vi "CRYRecall Editor.vi"() -> ()   [LabVIEW 2013]
uses:
  <vilib>/Utility/miscctls.llb/LVBoundsTypeDef.ctl
  Typedef Control/CRYRecall Cluster.ctl
  CRYProject/CRYProject Editor Global.vi
  CRYMainGlobal.vi
  CRYWindow/SubVI/CRYMain Sub Window Global.vi
  SubVI/CRYRecall Global.vi
  CRYStepSetup/CRYStepSetup Global.vi
panel:
  out "Recall Cluster Bk":T1={"Name"="Test for Signal [L]", "filepath"="Test for Signal [L]", "all or last"=0, "File Path Mode"=0, "Curve Names"=[], "format string"={"dB Format String out"="", "Lin Format String out"=""}, "Template"=[], "Axis"=0, "*.imp Path"=path "", "Filepath option"=0, "ML Value"=0.0, "user defined"="Test for Signal [L]", "Curves Selected?"=[], "Help"="", "Tab Value"=enum."Setting", "Selector"=0, "Use Default"=FALSE} {"Selector" items=["Space", "Underscores", "None"]; "Axis" scale=0.0..2.0; "Template" format="%#.0f"}
  in  "CurLibChange":bool caption="Add Lib"
  in  "Current Row":i32
  out "Auto Path":string
  out "Specify Path":string
  out "Auto Names":string[](array[string])
  out "Specify Names":string[](array[string])
  out "EndFlag":bool
  in  "Add Lib":bool
  in  "AddStep":bool
  in  "Table change":bool=TRUE
  out "Data type":string
  out "Row":u32
  in  "Board Tab":enum32{"Page 1"}(tab)
  in  "Cancel":bool caption="Apply"
  in  "OK":bool caption="Apply"
  in  "Main Tab":enum32{"Setting", "Help"}(tab)
  in  "Selector":i32(ring) caption="选择" items=["空格", "下划线", "无"]
  in  "Use default":bool caption="用户定义"
  in  "Format Value":bool
  out "single val":string
  in  "Select All":bool
  in  "Rename":bool
  in  "Clear2":bool
  in  "Add2":bool
  in  "Value":u16(ring) caption="值" items=["Max FSD Out Stimulus", "采集延迟 [Direct Out 1]", "采集延迟 [Direct Out 1] - P", "unity cal-in sens-in", "CRY33x Mic 1 sens-in", "CRY33x Mic 2 sens-in", "CRY33x Mic 3 sens-in", "CRY33x Mic 4 sens-in", "USB In L sens-in", "USB In R sens-in", "unity cal-out sens-out", "CRY602 Mouth 1 sens-out", "CRY602 Mouth 2 sens-out", "USB Out R sens-out", "Max FSD In [Direct In 1]", "2-采集延迟 [Direct Out 1]"]
  out "Template":string caption="模板"
  in  "User defined":string caption="用户定义"
  in  "Clear1":bool
  in  "Add1":bool
  in  "File Path Mode":u16(slide)
  in  "Recall Curve":u16(slide) caption="调用:"
  out "Recalled Curves":bool caption="调用曲线"
  out "File Path Information":bool caption="文件路径信息"
  in  "Base Path":path caption="基地路径"
  in  "Path Info":u16(slide)
  in  "filename constr":i32(listbox)=-1 caption="结构"
  in  ".imp Path":path caption=".imp file"
  in  "Names Control":string[][](table) caption="调用的曲线或结果名字"
  in  "Sel_1":bool
  in  "Sel_2":bool
  in  "Sel_3":bool
  in  "Sel_5":bool
  in  "Sel_4":bool
  in  "Sel_6":bool
  in  "Axis":u16(slide) caption="轴" scale=0.0..2.0
  in  "Help":string
  in  "Apply":bool
  in  "Load...":bool caption="Apply"
  in  "Save As...":bool caption="Apply"
  in  "Revert":bool caption="Apply"
  in  "Temp":u16[](array[numeric])
  in  "Hardware In":string
  in  "Calibration In":string
  in  "Channel":i32=1
  out "Set up Out":string
  in  "Set up In":string
  in  "stop":bool
  in  "Load Test":bool=TRUE
  in  "Recall Cluster":T1={"Name"="Test for Signal [L]", "filepath"="Test for Signal [L]", "all or last"=0, "File Path Mode"=0, "Curve Names"=[], "format string"={"dB Format String out"="", "Lin Format String out"=""}, "Template"=[], "Axis"=0, "*.imp Path"=path "", "Filepath option"=0, "ML Value"=0.0, "user defined"="Test for Signal [L]", "Curves Selected?"=[], "Help"="", "Tab Value"=enum."Setting", "Selector"=0, "Use Default"=FALSE} {"Selector" items=["Space", "Underscores", "None"]; "Axis" scale=0.0..2.0; "Template" format="%#.0f"}
  out "VIMiniumBound":T2
  in  "Proper VI No":i32
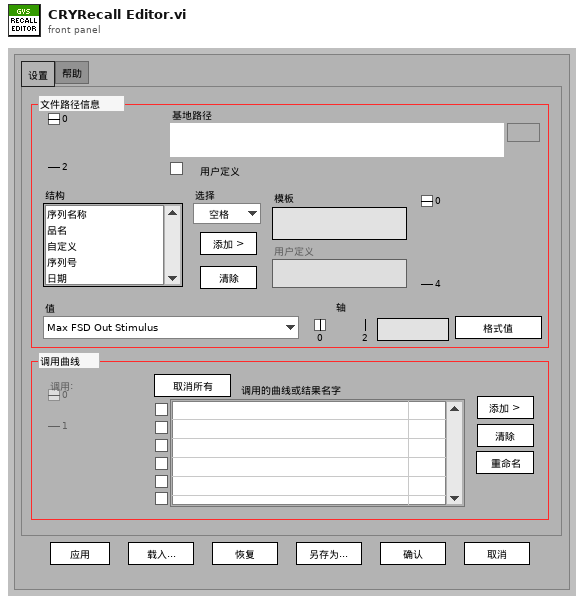
[diagram p1: front panel]
types:
  T1 = typedef "CRYRecall Cluster.ctl" = cluster{"Name":string, "filepath":string, "all or last":i32, "File Path Mode":u16, "Curve Names":string[], "format string":cluster{"dB Format String out":string, "Lin Format String out":string}, "Template":u16[], "Axis":u16, "*.imp Path":path, "Filepath option":i16, "ML Value":dbl, "user defined":string, "Curves Selected?":bool[], "Help":string, "Tab Value":enum32{"Setting", "Help"}, "Selector":i32, "Use Default":bool}
  T2 = typedef "LVBoundsTypeDef.ctl" = cluster{"Width":u32, "Height":u32}
  T3 = enum8{"Enabled", "Disabled", "Disabled and Grayed Out"}
  T4 = typedef "CRYStep.ctl" = cluster{"No.VI":i32, "Category":string, "StepName":string, "Seq setup flattened":string, "Comment":string, "Steps config.":bool[], "Jump config":i32[], "Start":dbl, "Increment":dbl, "Name":string, "Unit":string, "Y data":u16, "Y prefix":string, "Y dB ref":dbl, "Y unit":string, "Repeat State Array":cluster{"Start":dbl, "Increment":dbl, "Count":i32, "Num":i32}[]}
  T5 = typedef "LVRowAndColumnUnsignedTypeDef.ctl" = cluster{"Row":u32, "Column":u32}
  T6 = enum32{"English", "Chinese", "Korean", "Japanese", "Russian", "Chinese traditional"}
  T7 = enum16{"OK", "Yes", "YesNo", "YesNoCancel", "ReplaceAppend"}
  T8 = enum32{"existing file", "new file", "new or existing file", "existing dir", "new dir", "new or existing dir", "existing file (use LLBs)", "new file (use LLBs)", "new or existing file (use LLBs)", "new or existing file or directory (use LLBs)", "existing dir (use LLBs)", "new dir (use LLBs)", "new or existing dir (use LLBs)", "existing file or dir", "new file or dir", "new or existing file or dir", "existing file or dir (use LLBs)", "new file or dir (use LLBs)"}
  T9 = typedef "CRYData Cluster.ctl" = cluster{"Name":string, "Curve":cluster{"x":dbl, "y":dbl, "z":dbl}[], "X data":u16, "Y data":u16, "Z data":u16, "X axis":u16, "Y axis":u16, "Z axis":u16, "X unit":string, "Y unit":string, "Z unit":string, "X dB ref":dbl, "Y dB ref":dbl, "Z dB ref":dbl, "single val":bool, "protected":bool, "display X":bool, "display Y":bool, "display Z":bool, "Test Info":string, "Step No.":i32, "Plot Settings":cluster{"Color":u32, "Interpolation":u8, "Point Style":u8, "Line Style":u8, "Point Color":u32, "Line Width":u8, "Bar Plot Style":u8, "Fill To":i16}, "AutoProtect":bool}
  T10 = typedef "LVRowAndColumnTypeDef.ctl" = cluster{"Row":i32, "Column":i32}
  T11 = cluster{"Apply":bool, "Load Test":bool, bool, "Table change":bool, "Add Lib":bool, "OK":bool, "Cancel":bool}
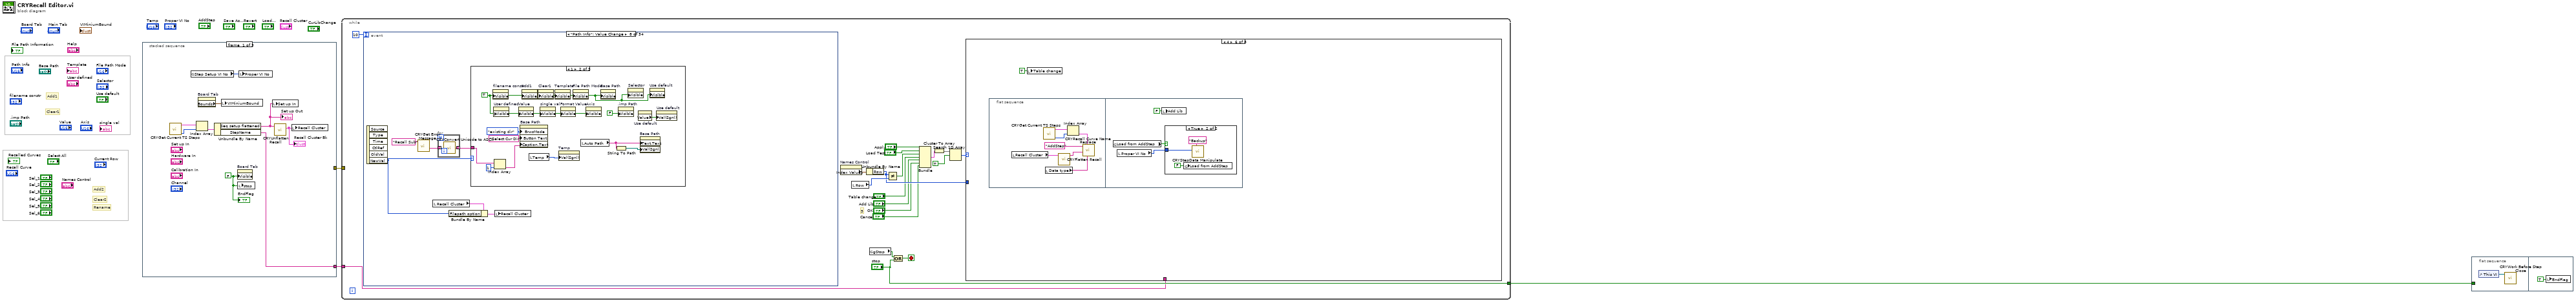
[diagram p0: block diagram]
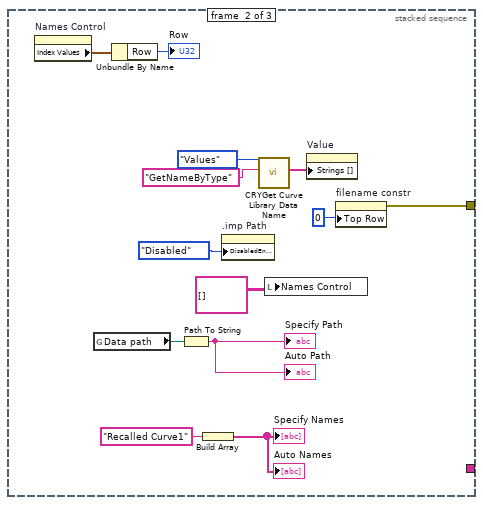
[diagram p2: hidden frame]
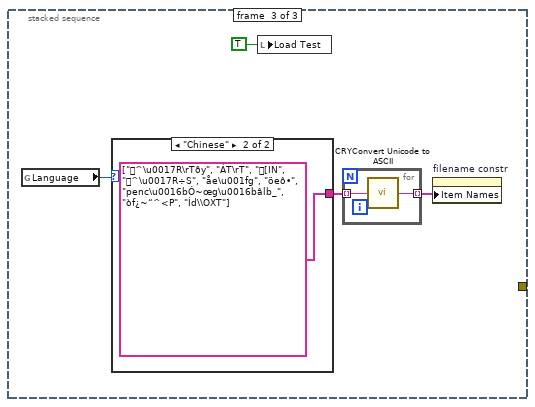
[diagram p3: hidden frame]
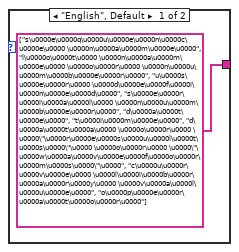
[diagram p4: hidden frame]
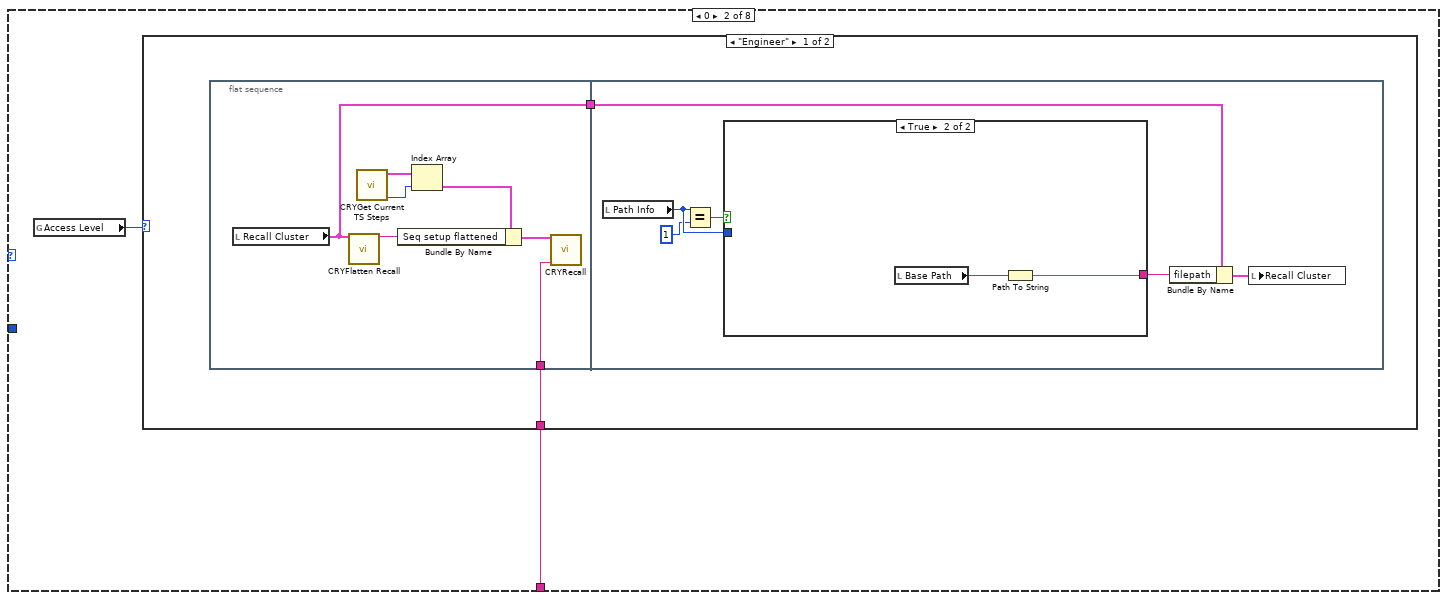
[diagram p6: hidden frame]
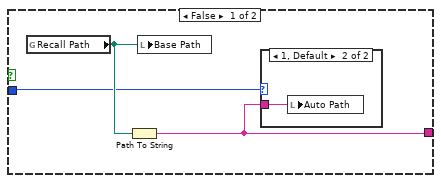
[diagram p7: hidden frame]
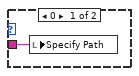
[diagram p8: hidden frame]
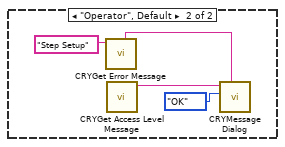
[diagram p9: hidden frame]
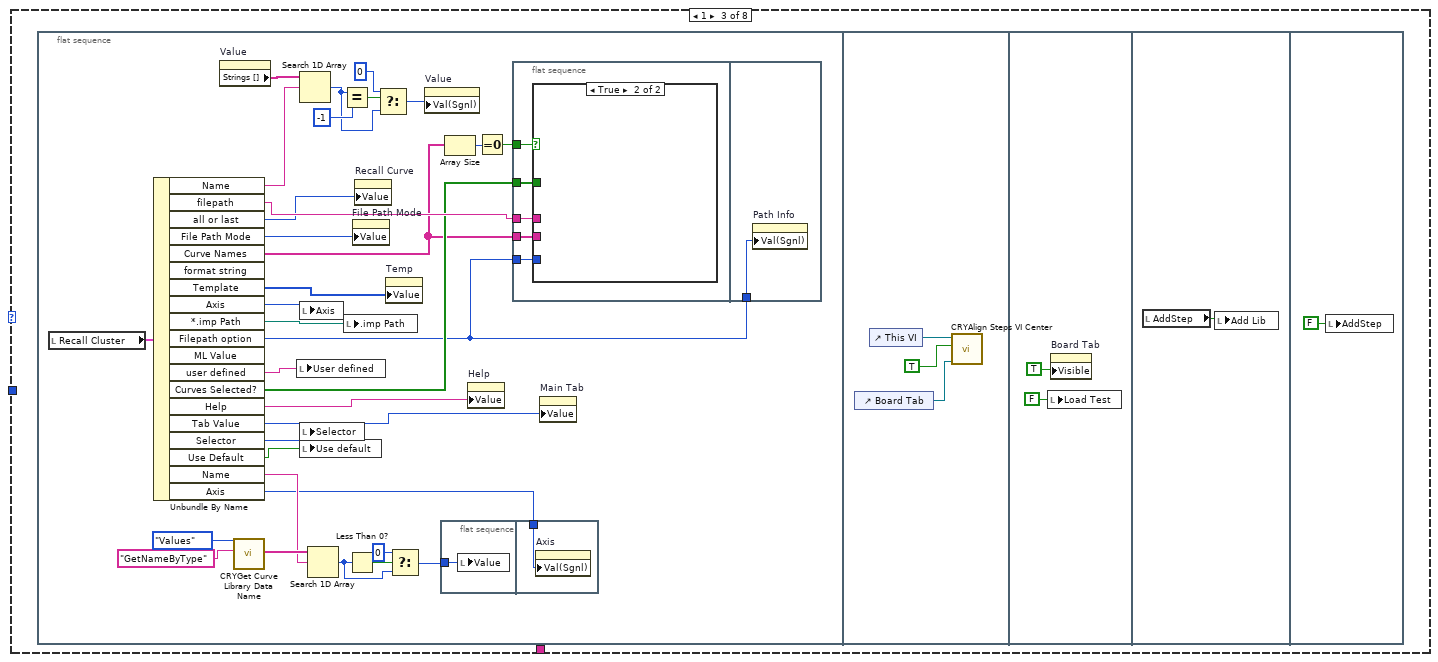
[diagram p10: hidden frame]
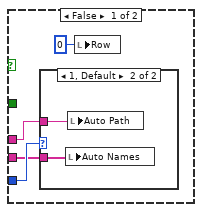
[diagram p11: hidden frame]
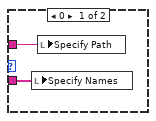
[diagram p12: hidden frame]
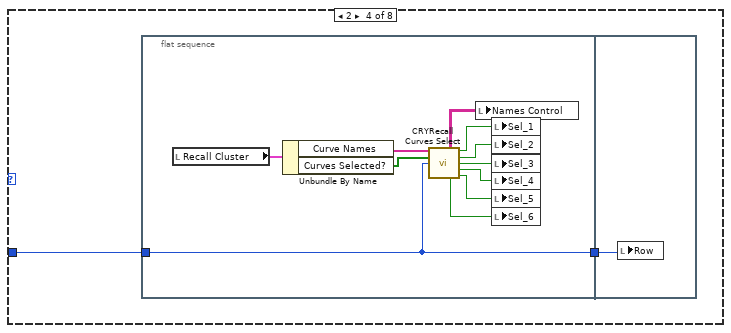
[diagram p13: hidden frame]
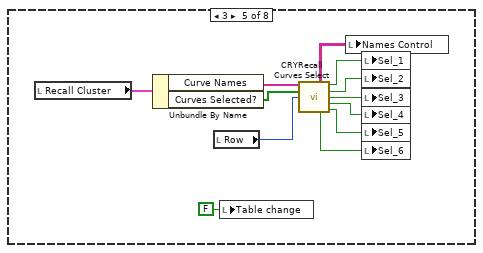
[diagram p14: hidden frame]
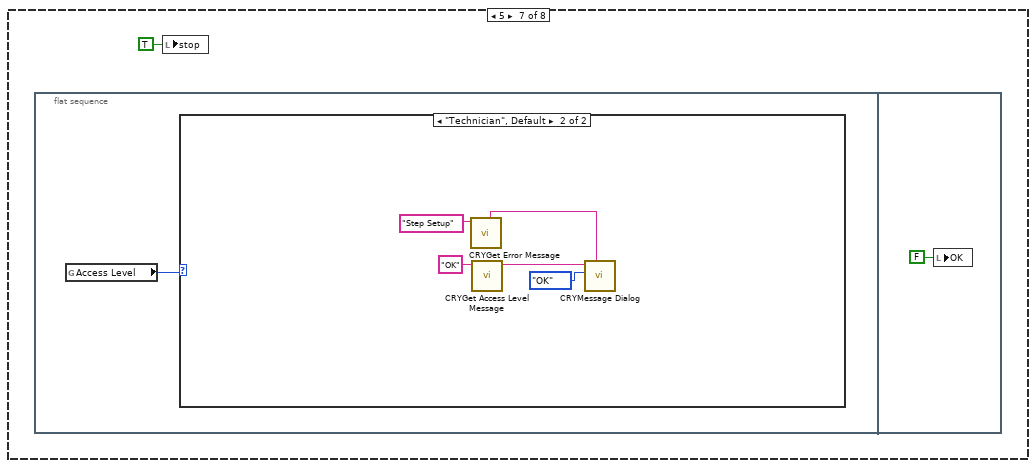
[diagram p16: hidden frame]
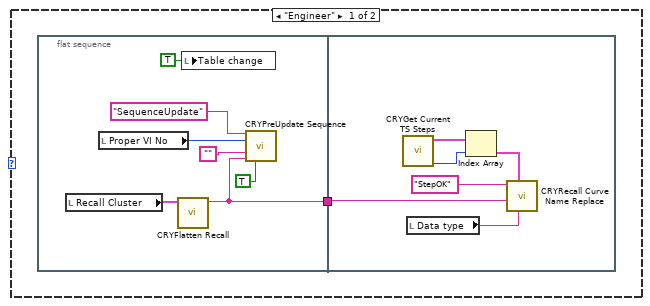
[diagram p17: hidden frame]
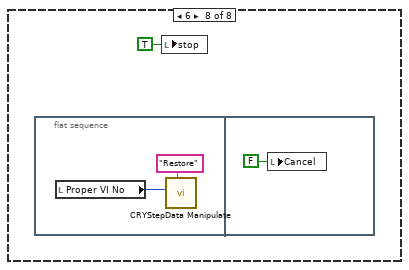
[diagram p18: hidden frame]
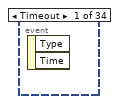
[diagram p19: hidden frame]
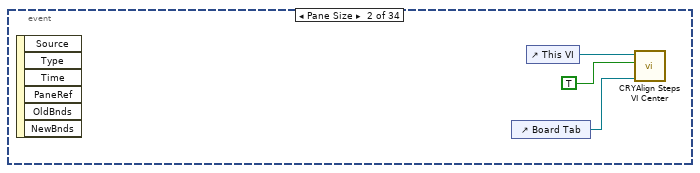
[diagram p20: hidden frame]
diagram:
  # "Rename"
  # "Clear2"
  # "Add2"
  # "Clear1"
  # "Add1"
  n1 = stacked-sequence {
    tunnel: [_ w13 _] -> w2
    tunnel: [w6 _ _] -> w1
    frame #0 {
      w4 = FALSE ("Visible")
      n2 = call "CRYGet Current TS Steps.vi"() -> ("SelectStepNumber in Tree"=w8:i32, "Steps"=w9:T4[])  [unwired: 7 in, 3 out]
      n3 = global read "CRYProject Editor Global.vi" "Step Setup VI No"() -> (w12:i32)
      n4 = Index Array(array=w9, index=w8) -> (element=w11:T4)
      n5 = property on="Board Tab" class="TabCtl (strict)"() -> ("Bounds"=w7:T2)  [unwired: 2 in, 2 out]
      n6 = Unbundle By Name(w11) -> ("Seq setup flattened"=w10:string, "StepName"=w6:string)
      "Set up Out" <- w10
      n7 = local write "VIMiniumBound"(w7) -> ()
      n8 = property on="Board Tab" class="TabCtl (strict)"("Visible"=w4) -> ()  [unwired: 2 in, 2 out]
      n9 = local write "stop"(w4) -> ()
      n10 = local write "Proper VI No"(w12) -> ()
      n11 = local write "Set up In"(w10) -> ()
      n12 = call "CRYUnflatten Recall.vi"("Flatten Recall"=w10) -> ("Recall setup"=w5:T1)  [unwired: 8 in, 2 out]
      "Recall Cluster Bk" <- w5
      n13 = local write "Recall Cluster"(w5) -> ()
      "EndFlag" <- w4
    }
    frame #1 {
      n14 = property on="Names Control" class="Tbl (strict)"() -> ("Index Values"=w21:T5)  [unwired: 2 in, 2 out]
      n15 = global read "CRYMainGlobal.vi" "Data path"() -> (w22:path)
      n16 = Unbundle By Name(w21) -> ("Row"=→"Row":u32)
      n17 = Path To String(path=w22) -> (string=→"Specify Path" →"Auto Path":string)
      n18 = Build Array("Recalled Curve1") -> (→"Specify Names" →"Auto Names":string[])
      n19 = property on=".imp Path" class="Path"("DisabledEnum"=T3."Disabled" ("Disabled")) -> ()  [unwired: 2 in, 2 out]
      n20 = call "CRYGet Curve Library Data Name.vi"("sAction"="GetNameByType", "Type"=enum16{"Curves", "Values", "Results", "WFM"}."Values") -> ("sNames"=w15:string[])  [unwired: 6 in, 3 out]
      n21 = local write "Names Control"(string[][] [] ("Item Names")) -> ()
      n22 = property on="Value" class="Ring (strict)"("Strings []"=w15) -> ()  [unwired: 2 in, 2 out]
      n23 = property on="filename constr" class="LstBox (strict)"("Top Row"=0 ("filename constr")) -> (error out=w13:errorcluster)  [unwired: 2 in, 1 out]
    }
    frame #2 {
      n24 = global read "CRYMainGlobal.vi" "Language"() -> (w28:T6)
      n25 = case shown="\"Chinese\"" w28 {
        tunnel: [string[] ["s\u0000e\u0000q\u0000u\u0000e\u0000n\u0000c\u0000e\u0000 \u0000n\u0000a\u0000m\u0000e\u0000", "l\u0000o\u0000t\u0000 \u0000n\u0000a\u0000m\u0000e\u0000 \u0000o\u0000r\u0000 \u0000n\u0000u\u0000m\u0000b\u0000e\u0000r\u0000", "u\u0000s\u0000e\u0000r\u0000 \u0000d\u0000e\u0000f\u0000i\u0000n\u0000e\u0000d\u0000", "s\u0000e\u0000r\u0000i\u0000a\u0000l\u0000 \u0000n\u0000u\u0000m\u0000b\u0000e\u0000r\u0000", "d\u0000a\u0000t\u0000e\u0000", "t\u0000i\u0000m\u0000e\u0000", "d\u0000a\u0000t\u0000a\u0000 \u0000o\u0000r\u0000 \u0000\"\u0000r\u0000e\u0000s\u0000u\u0000l\u0000t\u0000s\u0000\"\u0000 \u0000o\u0000r\u0000 \u0000\"\u0000w\u0000a\u0000v\u0000e\u0000f\u0000o\u0000r\u0000m\u0000s\u0000\"\u0000", "c\u0000u\u0000r\u0000v\u0000e\u0000 \u0000l\u0000i\u0000b\u0000r\u0000a\u0000r\u0000y\u0000 \u0000v\u0000a\u0000l\u0000u\u0000e\u0000", "o\u0000p\u0000e\u0000r\u0000a\u0000t\u0000o\u0000r\u0000"] string[] ["^\u0017R\rTðy", "ÁT\rT", "ꁚ[IN", "^\u0017R÷S", "åe\u001fg", "öeô•", "penc\u0016bÓ~œg\u0016bâlb_", "òf¿~“^<P", "Íd\\OXT"]] -> w27
        frame "English", Default {
        }
        frame "Chinese" {
        }
      }
      n26 = local write "Load Test"(TRUE ("Load Test")) -> ()
      n27 = for {
        tunnel: [w33] -> w26 mode=indexing
        tunnel: w27 -> [w32] mode=indexing
        n28 = call "CRYConvert Unicode to ASCII.vi"("Unicode"=w32) -> ("ASCII"=w33:string)  [unwired: 4 in]
      }
      n29 = property on="filename constr" class="LstBox (strict)"("Item Names"=w26) -> ()  [unwired: 2 in, 2 out]
    }
  }
  n30 = while {
    tunnel: ["stop"] -> w3
    tunnel: w2 -> [_]
    tunnel: w1 -> [w37]
    stop <- w46 stop-if-true
    # "5"
    n31 = event shown="[7] \"Path Info\": Value Change" {
      selector: _ -> [_ _ _ _ _ _ _ _ _ _ _ _ _ _ _ _ _ _ _ _ _ _ _ _ _ _ _ _ _ _ _ _ _ _]
      dyn-events: _ -> [_ _ _ _ _ _ _ _ _ _ _ _ _ _ _ _ _ _ _ _ _ _ _ _ _ _ _ _ _ _ _ _ _ _]
      timeout: 10 -> [_ _ _ _ _ _ _ _ _ _ _ _ _ _ _ _ _ _ _ _ _ _ _ _ _ _ _ _ _ _ _ _ _ _]
      event Timeout {
        n32 = event-data() -> ()  [unwired: 3 out]
      }
      event Pane Size {
        n33 = event-data() -> ()  [unwired: 7 out]
        n34 = control-ref of="Board Tab"() -> (w204:refnum<vi>)
        n35 = control-ref of="This VI"() -> (w203:refnum<vi>)
        n36 = call "CRYAlign Steps VI Center.vi"("Tab2"=w204, "Input/Output"=TRUE ("Preview"), "VIRef"=w203) -> ()  [unwired: 1 in, 8 out]
      }
      event "Load...": Value Change {
        n37 = event-data() -> ("CtlRef"=w206:refnum<vi>)  [unwired: 6 out]
        n38 = local read "Load Test"() -> (w208:bool)
        n39 = property class="Bool (strict)"(reference=w206, "Value"=FALSE) -> ()  [unwired: 1 in, 2 out]
        n40 = case shown="False" w208 {
          frame True {
          }
          frame False {
            n41 = global read "CRYMainGlobal.vi" "Steps path"() -> (w215:path)
            n42 = local read "Proper VI No"() -> (w210:i32)
            n43 = Build Path(base path=w215, name or relative path="CRYRecall") -> (appended path=w214:path)
            n44 = call "CRYStep Read.vi"("Category Name"="Recall", "Proper VI No"=w210, "Step File Path"=w214) -> ("status"=w212:bool, "selected path"=w209:path, "Flatten Step"=w211:string)  [unwired: 1 in, 3 out]
            n45 = case shown="True" w212 {
              tunnel: w211 -> [_ w218]
              tunnel: w210 -> [_ w219]
              tunnel: w209 -> [_ w217]
              frame False {
              }
              frame True {
                n46 = call "CRYUnflatten Recall.vi"("Flatten Recall"=w218) -> ("Error?"=w221:bool, "Recall setup"=w220:T1)  [unwired: 8 in, 1 out]
                n47 = case shown="False" w221 {
                  tunnel: w220 -> [w225 _]
                  tunnel: w219 -> [w224 _]
                  tunnel: w218 -> [w223 _]
                  tunnel: w217 -> [w222 _]
                  frame False {
                    n48 = flat-sequence {
                      tunnel: w225 -> [w237]
                      tunnel: w224 -> [w233]
                      tunnel: w223 -> [w232]
                      tunnel: w222 -> [w231]
                      frame #0 {
                        n49 = Strip Path(path=w231) -> (name=w226:string)  [unwired: 1 out]
                        n50 = local write "Recall Cluster"(w237) -> ()
                        n51 = Reverse String(1:w226) -> (0:w229:string)
                        n52 = Match Pattern(string=w229, regular expression="[.]") -> (after substring=w230:string)  [unwired: 4 out]
                        n53 = Reverse String(1:w230) -> (0:w227:string)
                        n54 = call "CRYPreUpdate Sequence.vi"("EventName"="Load", "StepName Arg3"=w227, "Proper VI No"=w233, "Project View Step Name Identifier Arg1"="", "Step flattened Arg2"=w232, "AllChangeFlg"=TRUE ("Name/Identifier")) -> ()  [unwired: 10 in]
                      }
                      frame #1 {
                        n55 = local write "Load Test"(TRUE ("Load Test")) -> ()
                      }
                    }
                  }
                  frame True {
                  }
                }
              }
            }
          }
        }
      }
      event "Save As...": Value Change {
        w243 = "Recall" ("Step File Name")
        n56 = event-data() -> ("CtlRef"=w239:refnum<vi>)  [unwired: 6 out]
        n57 = property class="Bool (strict)"(reference=w239, "Value"=FALSE) -> ()  [unwired: 1 in, 2 out]
        n58 = local read "Recall Cluster"() -> (w241:T1)
        n59 = call "CRYFlatten Recall.vi"("Recall"=w241) -> ("Recall flattened"=w242:string)  [unwired: 10 in]
        n60 = global read "CRYMainGlobal.vi" "Steps path"() -> (w245:path)
        n61 = Build Path(base path=w245, name or relative path="CRYRecall") -> (appended path=w244:path)
        n62 = local read "Proper VI No"() -> (w248:i32)
        n63 = call "CRYStep Write.vi"("StepIdentifier"="", "Default"=FALSE, "Proper VI No"=w248, "Category Name"=w243, "Step File Path"=w244, "Step flattened"=w242, "Step File Name"=w243) -> ()  [unwired: 1 in, 4 out]
      }
      event "Revert": Value Change {
        n64 = event-data() -> ("CtlRef"=w251:refnum<vi>)  [unwired: 6 out]
        n65 = property class="Bool (strict)"(reference=w251, "Value"=FALSE) -> ()  [unwired: 1 in, 2 out]
        n66 = flat-sequence {
          frame #0 {
            n67 = local read "Recall Cluster Bk"() -> (w252:T1)
            n68 = local write "Recall Cluster"(w252) -> ()
          }
          frame #1 {
            n69 = local write "Load Test"(TRUE ("Load Test")) -> ()
          }
        }
      }
      event Panel Close {
        n70 = event-data() -> ()  [unwired: 5 out]
        n71 = control-ref of="This VI"() -> (w255:refnum<vi>)
        n72 = local write "Cancel"(TRUE ("Cancel")) -> ()
        n73 = call "CRYWork Before Step Close.vi"("StepVI Ref"=w255) -> ()  [unwired: 11 in]
      }
      event "CurLibChange": Value Change {
        n74 = event-data() -> ()  [unwired: 7 out]
        n75 = call "CRYGet Curve Library Data Name.vi"("sAction"="GetNameByType", "Type"=enum16{"Curves", "Values", "Results", "WFM"}."Values") -> ("sNames"=w258:string[])  [unwired: 6 in, 3 out]
        n76 = property on="Value" class="Ring (strict)"("Strings []"=w258) -> ()  [unwired: 2 in, 2 out]
      }
      event "Path Info": Value Change {
        n77 = event-data() -> ("NewVal"=w261:u16)  [unwired: 6 out]
        n78 = call "CRYGet Error Message.vi"("Kind"="Recall Sub") -> ("Unicode Message Sub"=w260:string[])  [unwired: 5 in, 5 out]
        n79 = local read "Recall Cluster"() -> (w263:T1)
        n80 = for {
          tunnel: w260 -> [w266] mode=indexing
          tunnel: [w265] -> w259 mode=indexing
          n81 = call "CRYConvert Unicode to ASCII.vi"("Unicode"=w266) -> ("ASCII"=w265:string)  [unwired: 4 in]
        }
        n82 = Bundle By Name(cluster=w263, "Filepath option"=w261) -> (w262:T1)
        n83 = case shown="1" w261 {
          tunnel: w259 -> [w273 w283 w295]
          frame 0, Default {
            w269 = FALSE ("Visible")
            n84 = Index Array(array=w273, index=0) -> (element=w271:string)
            n85 = property on="Base Path" class="Path"("Visible"=TRUE) -> ()  [unwired: 2 in, 2 out]
            n86 = property on="filename constr" class="LstBox (strict)"("Visible"=w269) -> ()  [unwired: 2 in, 2 out]
            n87 = property on="File Path Mode" class="Slide (strict)"("Visible"=w269) -> ()  [unwired: 2 in, 2 out]
            n88 = local read "Specify Path"() -> (w268:string)
            n89 = property on="Value" class="Ring (strict)"("Visible"=w269) -> ()  [unwired: 2 in, 2 out]
            n90 = property on="Add1" class="Bool"("Visible"=w269) -> ()  [unwired: 2 in, 2 out]
            n91 = property on="Base Path" class="Path"("BrwsMode"=T8."existing file" ("Browse Options:Selection Mode"), "Button Text"="Open" ("Browse Options:Button Text"), "Caption.Text"=w271) -> ()  [unwired: 2 in, 2 out]
            n92 = String To Path(string=w268) -> (path=w274:path)
            n93 = property on="Template" class="Str"("Visible"=w269) -> ()  [unwired: 2 in, 2 out]
            n94 = property on="Clear1" class="Bool"("Visible"=w269) -> ()  [unwired: 2 in, 2 out]
            n95 = property on="Base Path" class="Path"("Text.Text"=w268, "Val(Sgnl)"=w274) -> ()  [unwired: 2 in, 2 out]
            n96 = property on="single val" class="Str"("Visible"=w269) -> ()  [unwired: 2 in, 2 out]
            n97 = property on="Axis" class="Slide (strict)"("Visible"=w269) -> ()  [unwired: 2 in, 2 out]
            n98 = property on="Format Value" class="Bool"("Visible"=w269) -> ()  [unwired: 2 in, 2 out]
            n99 = property on="User defined" class="Str"("Visible"=w269) -> ()  [unwired: 2 in, 2 out]
            n100 = property on="Selector" class="Ring (strict)"("Visible"=w269) -> ()  [unwired: 2 in, 2 out]
            n101 = property on=".imp Path" class="Path"("Visible"=FALSE) -> ()  [unwired: 2 in, 2 out]
            n102 = property on="Base Path" class="Path"("DisabledEnum"=T3."Enabled" ("Disabled")) -> ()  [unwired: 2 in, 2 out]
            n103 = property on="Use default" class="Bool (strict)"("Visible"=w269) -> ()  [unwired: 2 in, 2 out]
          }
          frame 1 {
            w280 = TRUE ("Visible")
            n104 = property on="filename constr" class="LstBox (strict)"("Visible"=w280) -> ()  [unwired: 2 in, 2 out]
            n105 = property on="User defined" class="Str"("Visible"=w280) -> ()  [unwired: 2 in, 2 out]
            n106 = Index Array(array=w283, index=1) -> (element=w281:string)
            n107 = property on="Value" class="Ring (strict)"("Visible"=w280) -> ()  [unwired: 2 in, 2 out]
            n108 = property on="Base Path" class="Path"("BrwsMode"=T8."existing dir" ("Browse Options:Selection Mode"), "Button Text"="Select Cur Dir" ("Browse Options:Button Text"), "Caption.Text"=w281) -> ()  [unwired: 2 in, 2 out]
            n109 = property on="Add1" class="Bool"("Visible"=w280) -> ()  [unwired: 2 in, 2 out]
            n110 = local read "Temp"() -> (w285:u16[])
            n111 = property on="Clear1" class="Bool"("Visible"=w280) -> ()  [unwired: 2 in, 2 out]
            n112 = property on="single val" class="Str"("Visible"=w280) -> ()  [unwired: 2 in, 2 out]
            n113 = property on="Template" class="Str"("Visible"=w280) -> ()  [unwired: 2 in, 2 out]
            n114 = property on="Temp" class="Arr (strict)"("Val(Sgnl)"=w285) -> ()  [unwired: 2 in, 2 out]
            n115 = property on="Format Value" class="Bool"("Visible"=w280) -> ()  [unwired: 2 in, 2 out]
            n116 = property on="File Path Mode" class="Slide (strict)"("Visible"=w280) -> ()  [unwired: 2 in, 2 out]
            n117 = local read "Auto Path"() -> (w279:string)
            n118 = property on="Axis" class="Slide (strict)"("Visible"=w280) -> ()  [unwired: 2 in, 2 out]
            n119 = property on="Base Path" class="Path"("Visible"=w280) -> ()  [unwired: 2 in, 2 out]
            n120 = String To Path(string=w279) -> (path=w284:path)
            n121 = property on=".imp Path" class="Path"("Visible"=FALSE) -> ()  [unwired: 2 in, 2 out]
            n122 = property on="Selector" class="Ring (strict)"("Visible"=w280) -> ()  [unwired: 2 in, 2 out]
            n123 = property on="Use default" class="Bool (strict)"() -> ("Value"=w278:bool)  [unwired: 2 in, 2 out]
            n124 = property on="Base Path" class="Path"("Text.Text"=w279, "Val(Sgnl)"=w284) -> ()  [unwired: 2 in, 2 out]
            n125 = property on="Use default" class="Bool (strict)"("Visible"=w280) -> ()  [unwired: 2 in, 2 out]
            n126 = property on="Use default" class="Bool (strict)"("Val(Sgnl)"=w278) -> ()  [unwired: 2 in, 2 out]
          }
          frame 2 {
            w291 = TRUE ("Visible")
            w299 = FALSE ("Visible")
            n127 = Index Array(array=w295, index=1) -> (element=w293:string)
            n128 = property on="filename constr" class="LstBox (strict)"("Visible"=w299) -> ()  [unwired: 2 in, 2 out]
            n129 = property on="User defined" class="Str"("Visible"=w299) -> ()  [unwired: 2 in, 2 out]
            n130 = property on="Base Path" class="Path"("BrwsMode"=T8."existing dir" ("Browse Options:Selection Mode"), "Button Text"="Select Cur Dir" ("Browse Options:Button Text"), "Caption.Text"=w293) -> ()  [unwired: 2 in, 2 out]
            n131 = property on="Value" class="Ring (strict)"("Visible"=w299) -> ()  [unwired: 2 in, 2 out]
            n132 = property on="Add1" class="Bool"("Visible"=w299) -> ()  [unwired: 2 in, 2 out]
            n133 = property on="Clear1" class="Bool"("Visible"=w299) -> ()  [unwired: 2 in, 2 out]
            n134 = property on="single val" class="Str"("Visible"=w299) -> ()  [unwired: 2 in, 2 out]
            n135 = property on="Selector" class="Ring (strict)"("Visible"=FALSE) -> ()  [unwired: 2 in, 2 out]
            n136 = property on="Template" class="Str"("Visible"=w299) -> ()  [unwired: 2 in, 2 out]
            n137 = property on="Format Value" class="Bool"("Visible"=w299) -> ()  [unwired: 2 in, 2 out]
            n138 = local read "Auto Path"() -> (w290:string)
            n139 = property on="Axis" class="Slide (strict)"("Visible"=w299) -> ()  [unwired: 2 in, 2 out]
            n140 = property on="File Path Mode" class="Slide (strict)"("Visible"=w291) -> ()  [unwired: 2 in, 2 out]
            n141 = property on=".imp Path" class="Path"("Visible"=w299) -> ()  [unwired: 2 in, 2 out]
            n142 = String To Path(string=w290) -> (path=w296:path)
            n143 = property on="Base Path" class="Path"("Visible"=w291) -> ()  [unwired: 2 in, 2 out]
            n144 = property on="Use default" class="Bool (strict)"() -> ("Value"=w289:bool)  [unwired: 2 in, 2 out]
            n145 = property on="Base Path" class="Path"("Text.Text"=w290, "Val(Sgnl)"=w296) -> ()  [unwired: 2 in, 2 out]
            n146 = property on="Use default" class="Bool (strict)"("Val(Sgnl)"=w289) -> ()  [unwired: 2 in, 2 out]
            n147 = property on="Use default" class="Bool (strict)"("Visible"=w291) -> ()  [unwired: 2 in, 2 out]
          }
        }
        n148 = local write "Recall Cluster"(w262) -> ()
      }
      event "Base Path": Value Change {
        n149 = event-data() -> ("OldVal"=w300:path, "NewVal"=w301:path)  [unwired: 5 out]
        n150 = stacked-sequence {
          tunnel: w301 -> [w303 _]
          tunnel: w300 -> [w304 _]
          frame #0 {
            n151 = Path To String(path=w303) -> (string=w308:string)
            n152 = File/Directory Info(path=w303) -> (error out=w330:errorcluster)  [unwired: 1 in, 6 out]
            n153 = global write "CRYRecall Global.vi" "Recall Path"(w303) -> ()
            n154 = global read "CRYMainGlobal.vi" "Language"() -> (w306:T6)
            n155 = Unbundle By Name(w330) -> ("status"=w320:bool)
            n156 = call <vilib>:"Get File Extension.vi"("file"=w303) -> ("lowercase file extension"=w310:string)  [unwired: 7 in, 3 out]
            n157 = Not Equal?(x=w303, y=w304) -> (x != y?=w302:bool)
            n158 = Strip Path(path=w303) -> (stripped path=w324:path)  [unwired: 1 out]
            n159 = case shown="\"English\", Default" w306 {
              tunnel: ["R\u0000e\u0000c\u0000a\u0000l\u0000l\u0000e\u0000d\u0000 \u0000C\u0000u\u0000r\u0000v\u0000e\u00001\u0000" ("Table") "\u0003Œ(u‡eöNòf¿~1\u0000" ("Label.Text")] -> w307
              frame "English", Default {
              }
              frame "Chinese" {
              }
            }
            n160 = Not(x=w320) -> (.not. x?=w319:bool)
            n161 = Empty String/Path?(string/path=w324) -> (empty?=w322:bool)
            n162 = local read "Path Info"() -> (w309:u16)
            n163 = local read "Recall Cluster"() -> (w323:T1)
            n164 = Not(x=w322) -> (.not. x?=w321:bool)
            n165 = Equal?(x="txt", y=w310) -> (x = y?=w317:bool)
            n166 = Equal?(x="dat", y=w310) -> (x = y?=w316:bool)
            n167 = Equal?(x="res", y=w310) -> (x = y?=w315:bool)
            n168 = Equal?(x="wfm", y=w310) -> (x = y?=w314:bool)
            n169 = Equal?(x="wav", y=w310) -> (x = y?=w311:bool)
            n170 = Compound Arithmetic op=OR(w317, w316, w315, w314, w311) -> (w325:bool)
            n171 = call "CRYConvert Unicode to ASCII.vi"("Unicode"=w307) -> ("ASCII"=w305:string)  [unwired: 4 in]
            n172 = Compound Arithmetic op=AND(w321, w319, w325) -> (w318:bool)
            n173 = case shown="1, Default" w309 {
              tunnel: w308 -> [w333 w334]
              frame 0 {
                n174 = local write "Specify Path"(w333) -> ()
              }
              frame 1, Default {
                n175 = local write "Auto Path"(w334) -> ()
              }
            }
            n176 = case shown="0, Default" w309 {
              tunnel: w308 -> [w351 _]
              tunnel: w323 -> [w350 w406]
              tunnel: [w349 w405] -> w313
              tunnel: w318 -> [w348 _]
              tunnel: w317 -> [w347 _]
              tunnel: w316 -> [w346 _]
              tunnel: w315 -> [w345 _]
              tunnel: w314 -> [w344 _]
              tunnel: w311 -> [w343 _]
              tunnel: w305 -> [w342 w401]
              tunnel: w302 -> [w341 _]
              frame 0, Default {
                # "Specify"
                n177 = case shown="True" w348 {
                  tunnel: w351 -> [_ w370]
                  tunnel: w350 -> [w356 w368]
                  tunnel: [w354 w367] -> w349
                  tunnel: w347 -> [_ w364]
                  tunnel: w346 -> [_ w363]
                  tunnel: w345 -> [_ w362]
                  tunnel: w344 -> [_ w361]
                  tunnel: w343 -> [_ w360]
                  tunnel: w342 -> [w353 w358]
                  tunnel: w341 -> [_ w357]
                  frame False {
                    # "file = no"
                    n178 = Build Array(w353) -> (w355:string[])
                    n179 = local write "Specify Names"(w355) -> ()
                    n180 = Bundle By Name(cluster=w356, "Curve Names"=w355, "Curves Selected?"=bool[] [TRUE]) -> (w354:T1)
                  }
                  frame True {
                    # "file = ok"
                    n181 = call "CRYCurves read & count.vi"("Last curve only (F)"=FALSE, "Data file path"=w370) -> ("Curve or Result names"=w365:string[], "Canceled"=w369:bool, "Data curves array"=w366:string[])  [unwired: 6 in, 1 out]
                    n182 = case shown="False" w369 {
                      tunnel: w365 -> [w372 _]
                      tunnel: w368 -> [w384 w400]
                      tunnel: [w383 w398] -> w367
                      tunnel: w366 -> [_ _]
                      tunnel: w364 -> [w379 _]
                      tunnel: w363 -> [w378 _]
                      tunnel: w362 -> [w377 _]
                      tunnel: w361 -> [w376 _]
                      tunnel: w360 -> [w373 _]
                      tunnel: w358 -> [_ w397]
                      tunnel: w357 -> [w371 _]
                      frame False {
                        # "data = ok"
                        n183 = Bundle(w379, w378, w377, w376, w373) -> (w380:cluster{bool, bool, bool, bool, bool})  [unwired: 1 out]
                        n184 = Cluster To Array(cluster=w380) -> (array=w381:bool[])
                        n185 = Search 1D Array(1D array=w381, element=TRUE) -> (index of element=w375:i32)  [unwired: 1 out]
                        n186 = case shown="False" w371 {
                          tunnel: w384 -> [w385 w391]
                          tunnel: [w385 w390] -> w383
                          tunnel: w372 -> [_ w386]
                          frame False {
                          }
                          frame True {
                            n187 = local write "Specify Names"(w386) -> ()
                            n188 = Array Size(array=w386) -> (size(s)=w389:i32)
                            n189 = Initialize Array(TRUE ("element"), w389) -> (w387:bool[])
                            n190 = Bundle By Name(cluster=w391, "Curves Selected?"=w387, "Curve Names"=w386) -> (w390:T1)
                          }
                        }
                        n191 = case shown="3, 4" w375 {
                          tunnel: ["Data" ("Data type") "Result" ("Data type") "Waveform" ("Data type")] -> w374
                          frame 0, 1, Default {
                          }
                          frame 2 {
                          }
                          frame 3, 4 {
                          }
                        }
                        "Data type" <- w374
                      }
                      frame True {
                        # "data = empty"
                        n192 = local write "Data type"("Data" ("t")) -> ()
                        n193 = Build Array(w397) -> (w399:string[])
                        n194 = local write "Specify Names"(w399) -> ()
                        n195 = Bundle By Name(cluster=w400, "Curve Names"=w399, "Curves Selected?"=bool[] [TRUE]) -> (w398:T1)
                      }
                    }
                  }
                }
              }
              frame 1, 2 {
                # "Automatic, Prompt"
                n196 = Unbundle By Name(w406) -> ("Curve Names"=w403:string[])
                n197 = Array Size(array=w403) -> (size(s)=w404:i32)
                n198 = Equal To 0?(x=w404) -> (x = 0?=w402:bool)
                n199 = case shown="True" w402 {
                  tunnel: w406 -> [w407 w414]
                  tunnel: [w407 w413] -> w405
                  tunnel: w401 -> [_ w408]
                  frame False {
                  }
                  frame True {
                    n200 = Build Array(w408) -> (w409:string[])
                    n201 = Array Size(array=w409) -> (size(s)=w412:i32)
                    n202 = local write "Auto Names"(w409) -> ()
                    n203 = Initialize Array(TRUE ("element"), w412) -> (w410:bool[])
                    n204 = Bundle By Name(cluster=w414, "Curve Names"=w409, "Curves Selected?"=w410) -> (w413:T1)
                  }
                }
              }
            }
            n205 = case shown="False" w311 {
              frame False {
                n206 = property on="Recall Curve" class="Slide (strict)"("DisabledEnum"=T3."Enabled" ("Disabled")) -> ()  [unwired: 2 in, 2 out]
              }
              frame True {
                n207 = property on="Recall Curve" class="Slide (strict)"("DisabledEnum"=T3."Disabled and Grayed Out" ("Disabled"), "Value"=u16 0 ("index")) -> ()  [unwired: 2 in, 2 out]
              }
            }
            n208 = flat-sequence {
              tunnel: w308 -> [w337]
              tunnel: w313 -> [w336]
              frame #0 {
                n209 = Bundle By Name(cluster=w336, "filepath"=w337) -> (w335:T1)
                n210 = local write "Recall Cluster"(w335) -> ()
              }
            }
          }
          frame #1 {
            n211 = local read "Path Info"() -> (w415:u16)
            n212 = case shown="0, Default" w415 {
              frame 0, Default {
                n213 = local read "Recall Curve"() -> (w416:u16)
                n214 = property on="Recall Curve" class="Slide (strict)"("Val(Sgnl)"=w416) -> ()  [unwired: 2 in, 2 out]
              }
              frame 1, 2 {
                n215 = local read "File Path Mode"() -> (w417:u16)
                n216 = property on="File Path Mode" class="Slide (strict)"("Val(Sgnl)"=w417) -> ()  [unwired: 2 in, 2 out]
              }
            }
          }
        }
      }
      event "Recall Curve": Value Change {
        n217 = event-data() -> ("OldVal"=w418:u16, "NewVal"=w419:u16)  [unwired: 5 out]
        n218 = case shown="0, Default" w419 {
          frame 0, Default {
            w444 = T3."Enabled" ("Disabled")
            n219 = property on="Sel_1" class="Bool (strict)"("DisabledEnum"=w444) -> ()  [unwired: 2 in, 2 out]
            n220 = property on="Sel_2" class="Bool (strict)"("DisabledEnum"=w444) -> ()  [unwired: 2 in, 2 out]
            n221 = property on="Sel_3" class="Bool (strict)"("DisabledEnum"=w444) -> ()  [unwired: 2 in, 2 out]
            n222 = property on="Select All" class="Bool (strict)"("Value"=FALSE ("Select"), "DisabledEnum"=w444, "Key Focus"=TRUE) -> ()  [unwired: 2 in, 2 out]
            n223 = property on="Sel_4" class="Bool (strict)"("DisabledEnum"=w444) -> ()  [unwired: 2 in, 2 out]
            n224 = property on="Sel_5" class="Bool (strict)"("DisabledEnum"=w444) -> ()  [unwired: 2 in, 2 out]
            n225 = property on="Sel_6" class="Bool (strict)"("DisabledEnum"=w444) -> ()  [unwired: 2 in, 2 out]
          }
          frame 1 {
            w447 = T3."Disabled and Grayed Out" ("Disabled")
            n226 = property on="Sel_1" class="Bool (strict)"("DisabledEnum"=w447) -> ()  [unwired: 2 in, 2 out]
            n227 = property on="Sel_2" class="Bool (strict)"("DisabledEnum"=w447) -> ()  [unwired: 2 in, 2 out]
            n228 = property on="Sel_3" class="Bool (strict)"("DisabledEnum"=w447) -> ()  [unwired: 2 in, 2 out]
            n229 = property on="Select All" class="Bool (strict)"("Value"=TRUE ("Select"), "DisabledEnum"=w447) -> ()  [unwired: 2 in, 2 out]
            n230 = property on="Sel_4" class="Bool (strict)"("DisabledEnum"=w447) -> ()  [unwired: 2 in, 2 out]
            n231 = property on="Sel_5" class="Bool (strict)"("DisabledEnum"=w447) -> ()  [unwired: 2 in, 2 out]
            n232 = property on="Sel_6" class="Bool (strict)"("DisabledEnum"=w447) -> ()  [unwired: 2 in, 2 out]
          }
        }
        n233 = Not Equal?(x=w418, y=w419) -> (x != y?=w420:bool)
        n234 = case shown="False" w420 {
          tunnel: w419 -> [_ w422]
          frame False {
            n235 = local write "Table change"(TRUE ("Table change")) -> ()
          }
          frame True {
            n236 = flat-sequence {
              tunnel: w422 -> [w428]
              frame #0 {
                n237 = local read "Path Info"() -> (w423:u16)
                n238 = case shown="0" w423 {
                  tunnel: [w430 w431] -> w424
                  frame 0 {
                    n239 = local read "Specify Names"() -> (w430:string[])
                  }
                  frame 1, Default {
                    n240 = local read "Auto Names"() -> (w431:string[])
                  }
                }
                n241 = case shown="0, Default" w428 {
                  tunnel: w424 -> [w433 w438]
                  tunnel: [w433 w437] -> w426
                  tunnel: [w432 w436] -> w425
                  frame 0, Default {
                    n242 = Array Size(array=w433) -> (size(s)=w434:i32)
                    n243 = Initialize Array(TRUE ("Sel_6"), w434) -> (w432:bool[])
                  }
                  frame 1 {
                    n244 = Array Size(array=w438) -> (size(s)=w440:i32)
                    n245 = Decrement(x=w440) -> (x-1=w439:i32)
                    n246 = Build Array(TRUE ("Sel_6")) -> (w436:bool[])
                    n247 = Index Array(array=w438, index=w439) -> (element=w441:string)
                    n248 = Build Array(w441) -> (w437:string[])
                  }
                }
                n249 = local read "Recall Cluster"() -> (w429:T1)
                n250 = Bundle By Name(cluster=w429, "Curve Names"=w426, "Curves Selected?"=w425, "all or last"=w428) -> (w427:T1)
                n251 = local write "Recall Cluster"(w427) -> ()
              }
              frame #1 {
                n252 = local write "Table change"(TRUE ("Table change")) -> ()
              }
            }
          }
        }
      }
      event "Temp": Value Change {
        n253 = event-data() -> ("NewVal"=w453:u16[])  [unwired: 6 out]
        n254 = global read "CRYMainGlobal.vi" "Language"() -> (w449:T6)
        n255 = case shown="\"Chinese\"" w449 {
          tunnel: [string[] ["<\u0000s\u0000e\u0000q\u0000>\u0000", "<\u0000l\u0000o\u0000t\u0000>\u0000", "<\u0000u\u0000s\u0000e\u0000r\u0000>\u0000", "<\u0000s\u0000n\u0000>\u0000", "<\u0000d\u0000a\u0000t\u0000e\u0000>\u0000", "<\u0000t\u0000i\u0000m\u0000e\u0000>\u0000", "<\u0000d\u0000 \u0000o\u0000r\u0000 \u0000r\u0000>\u0000", "<\u0000c\u0000l\u0000v\u0000a\u0000l\u0000>\u0000", "<\u0000o\u0000p\u0000e\u0000r\u0000>\u0000"] string[] ["<\u0000^\u0017R\rTðy>\u0000", "<\u0000ÁT\rT>\u0000", "<\u0000ꁚ[IN>\u0000", "<\u0000^\u0017R÷S>\u0000", "<\u0000åe\u001fg>\u0000", "<\u0000öeô•>\u0000", "<\u0000penc\u0016bÓ~œg\u0016bâl>\u0000", "<\u0000òf¿~“^<P>\u0000", "<\u0000Íd\\OXT>\u0000"]] -> w451
          frame "English", Default {
          }
          frame "Chinese" {
          }
        }
        n256 = local read "Path Info"() -> (w457:u16)
        n257 = for {
          tunnel: [w459] -> w450 mode=indexing
          tunnel: w451 -> [w458] mode=indexing
          n258 = call "CRYConvert Unicode to ASCII.vi"("Unicode"=w458) -> ("ASCII"=w459:string)  [unwired: 4 in]
        }
        n259 = Equal?(x=w457, y=u16 1) -> (x = y?=w455:bool)
        n260 = case shown="True" w455 {
          tunnel: w453 -> [_ w464]
          tunnel: w450 -> [_ w463]
          frame False {
          }
          frame True {
            w465 = ""
            w469 = T3."Disabled and Grayed Out" ("Disabled")
            w468 = T3."Enabled" ("Disabled")
            n261 = Search 1D Array(1D array=w464, element=u16 2) -> (index of element=w476:i32)  [unwired: 1 in]
            n262 = Search 1D Array(1D array=w464, element=u16 7) -> (index of element=w473:i32)  [unwired: 1 in]
            n263 = Equal?(x=w473, y=-1) -> (x = y?=w470:bool)
            n264 = Equal?(x=w476, y=-1) -> (x = y?=w471:bool)
            n265 = for {
              shift-right: [w478] -> w462
              shift-left: w465 -> [w482]
              tunnel: w465 -> [w483]
              tunnel: w464 -> [w481] mode=indexing
              tunnel: w463 -> [w480]
              n266 = Index Array(array=w480, index=w481) -> (element=w479:string)
              n267 = Empty String/Path?(string/path=w482) -> (empty?=w486:bool)
              n268 = Select(t=w483, s=w486, f=" ") -> (s? t:f=w484:string)
              n269 = Concatenate Strings(w482, w484, w479) -> (w478:string)
            }
            n270 = Select(t=w469, s=w471, f=w468) -> (s? t:f=w467:T3)
            n271 = Select(t=w469, s=w470, f=w468) -> (s? t:f=w466:T3)
            n272 = property on="Value" class="Ring (strict)"("DisabledEnum"=w466) -> ()  [unwired: 2 in, 2 out]
            n273 = property on="User defined" class="Str"("DisabledEnum"=w467) -> ()  [unwired: 2 in, 2 out]
            n274 = property on="single val" class="Str"("DisabledEnum"=w466) -> ()  [unwired: 2 in, 2 out]
            n275 = property on="Format Value" class="Bool"("DisabledEnum"=w466) -> ()  [unwired: 2 in, 2 out]
            n276 = local write "Template"(w462) -> ()
            n277 = property on="Axis" class="Slide (strict)"("DisabledEnum"=w466) -> ()  [unwired: 2 in, 2 out]
          }
        }
        n278 = local read "Recall Cluster"() -> (w454:T1)
        n279 = Bundle By Name(cluster=w454, "Template"=w453) -> (w452:T1)
        n280 = local write "Recall Cluster"(w452) -> ()
      }
      event "File Path Mode": Value Change {
        n281 = event-data() -> ("NewVal"=w493:u16)  [unwired: 6 out]
        n282 = Equal?(x=w493, y=u16 2) -> (x = y?=w491:bool)
        n283 = local read "Recall Cluster"() -> (w494:T1)
        n284 = Bundle By Name(cluster=w494, "File Path Mode"=w493) -> (w492:T1)
        n285 = Select(t=T3."Disabled and Grayed Out" ("Disabled"), s=w491, f=T3."Enabled" ("Disabled")) -> (s? t:f=w488:T3)
        n286 = local write "Table change"(TRUE ("Table change")) -> ()
        n287 = property on="Recall Curve" class="Slide (strict)"("DisabledEnum"=w488) -> ()  [unwired: 2 in, 2 out]
        n288 = local write "Recall Cluster"(w492) -> ()
      }
      event "Use default": Value Change {
        n289 = event-data() -> ("NewVal"=w498:bool)  [unwired: 6 out]
        n290 = local read "Recall Cluster"() -> (w503:T1)
        n291 = Bundle By Name(cluster=w503, "Use Default"=w498) -> (w502:T1)
        n292 = local write "Recall Cluster"(w502) -> ()
        n293 = Select(t=T3."Disabled and Grayed Out" ("Disabled"), s=w498, f=T3."Enabled" ("Disabled")) -> (s? t:f=w500:T3)
        n294 = property on="Base Path" class="Path"("DisabledEnum"=w500) -> ()  [unwired: 2 in, 2 out]
        n295 = local read "Path Info"() -> (w497:u16)
        n296 = case shown="1, Default" w497 {
          tunnel: w498 -> [_ w507]
          tunnel: [w504 w506] -> w496
          frame 0 {
            n297 = local read "Specify Path"() -> (w505:string)
            n298 = String To Path(string=w505) -> (path=w504:path)
          }
          frame 1, Default {
            n299 = case shown="False" w507 {
              tunnel: [w508 w510] -> w506
              frame False {
                n300 = local read "Auto Path"() -> (w509:string)
                n301 = String To Path(string=w509) -> (path=w508:path)
              }
              frame True {
                n302 = global read "CRYMainGlobal.vi" "Data path"() -> (w510:path)
              }
            }
          }
        }
        n303 = property on="Base Path" class="Path"("Value"=w496) -> ()  [unwired: 2 in, 2 out]
      }
      event "Selector": Value Change {
        n304 = event-data() -> ("NewVal"=w511:i32)  [unwired: 6 out]
        n305 = local read "Recall Cluster"() -> (w513:T1)
        n306 = Bundle By Name(cluster=w513, "Selector"=w511) -> (w512:T1)
        n307 = local write "Recall Cluster"(w512) -> ()
      }
      event "Add1": Value Change {
        n308 = event-data() -> ()  [unwired: 7 out]
        n309 = local read "filename constr"() -> (w514:i32)
        n310 = case shown="True" "Add1" {
          tunnel: string[] ["<seq>", "<lot>", "<user>", "<sn>", "<date>", "<time>", "<d or r>", "<clval>", "<oper>"] -> [_ w517]
          tunnel: w514 -> [_ w518]
          frame False {
          }
          frame True {
            n311 = Greater Or Equal?(x=w518, y=0) -> (x >= y?=w519:bool)
            n312 = case shown="False" w519 {
              tunnel: w518 -> [_ w529]
              tunnel: w517 -> [_ w533]
              frame False {
                n313 = call "CRYGet Error Message.vi"("Error No"=0, "Kind"="Recall") -> ("Message"=w523:string, "Window Title"=w522:string)  [unwired: 4 in, 4 out]
                n314 = call "CRYMessage Dialog.vi"("Window Title"=w522, "YesNoCancel"=T7."OK", "Message Content"=w523) -> ()  [unwired: 7 in, 2 out]
              }
              frame True {
                n315 = local read "Template"() -> (w531:string)
                n316 = local read "Temp"() -> (w530:u16[])
                n317 = Index Array(array=w533, index=w529) -> (element=w538:string)
                n318 = Build Array (concatenate)(w530, w529) -> (w527:i32[])
                n319 = Empty String/Path?(string/path=w531) -> (empty?=w536:bool)
                n320 = Select(t="", s=w536, f=" ") -> (s? t:f=w534:string)
                n321 = local read "Recall Cluster"() -> (w528:T1)
                n322 = Concatenate Strings(w531, w534, w538) -> (w532:string)
                n323 = Bundle By Name(cluster=w528, "Template"=w527) -> (w526:T1)
                n324 = property on="Temp" class="Arr (strict)"("Val(Sgnl)"=w527) -> ()  [unwired: 2 in, 2 out]
                n325 = local write "Template"(w532) -> ()
                n326 = local write "Recall Cluster"(w526) -> ()
              }
            }
          }
        }
      }
      event "Clear1": Value Change {
        n327 = event-data() -> ()  [unwired: 7 out]
        n328 = case shown="True" "Clear1" {
          frame False {
          }
          frame True {
            n329 = local write "Template"("") -> ()
            n330 = property on="Temp" class="Arr (strict)"("Val(Sgnl)"=u16[] [] ("Value (Signaling)")) -> ()  [unwired: 2 in, 2 out]
          }
        }
      }
      event "Axis": Value Change {
        n331 = event-data() -> ("NewVal"=w552:u16)  [unwired: 6 out]
        n332 = property on="Value" class="Ring (strict)"() -> ("Strings []"=w543:string[])  [unwired: 2 in, 2 out]
        n333 = local read "Value"() -> (w544:u16)
        n334 = Index Array(array=w543, index=w544) -> (element=w545:string)
        n335 = local read "Recall Cluster"() -> (w550:T1)
        n336 = call "CRYGet Curve Library One Data .vi"("Data Name"=w545, "Type"=enum16{"Curves", "Values", "Results", "WFM"}."Values") -> ("Value"=w542:T9)  [unwired: 3 in, 6 out]
        n337 = Unbundle By Name(w542) -> ("Curve"=w554:cluster{"x":dbl, "y":dbl, "z":dbl}[])
        n338 = Bundle By Name(cluster=w550, "Axis"=w552) -> (w551:T1)
        n339 = Unbundle By Name(w550) -> ("format string.Lin Format String out"=w549:string)
        n340 = local write "Recall Cluster"(w551) -> ()
        n341 = Index Array(array=w554) -> (element=w553:cluster{"x":dbl, "y":dbl, "z":dbl})  [unwired: 1 in]
        n342 = case shown="0, Default" w552 {
          tunnel: w553 -> [w556 w558 w560]
          tunnel: [w555 w557 w559] -> w548
          frame 0, Default {
            n343 = Unbundle By Name(w556) -> ("x"=w555:dbl)
          }
          frame 1 {
            n344 = Unbundle By Name(w558) -> ("y"=w557:dbl)
          }
          frame 2 {
            n345 = Unbundle By Name(w560) -> ("z"=w559:dbl)
          }
        }
        n346 = call "CRYGet Formated String Value.vi"("Value"=w548, "Flattened Format String"=w549) -> ("Unflattened Format string"=w547:string)  [unwired: 9 in]
        n347 = local write "single val"(w547) -> ()
      }
      event "Value": Value Change {
        n348 = event-data() -> ("NewVal"=w566:u16)  [unwired: 6 out]
        n349 = property on="Value" class="Ring (strict)"() -> ("Strings []"=w565:string[])  [unwired: 2 in, 2 out]
        n350 = Index Array(array=w565, index=w566) -> (element=w563:string)
        n351 = local read "Recall Cluster"() -> (w564:T1)
        n352 = local read "Axis"() -> (w562:u16)
        n353 = Bundle By Name(cluster=w564, "Name"=w563) -> (w561:T1)
        n354 = property on="Axis" class="Slide (strict)"("Val(Sgnl)"=w562) -> ()  [unwired: 2 in, 2 out]
        n355 = local write "Recall Cluster"(w561) -> ()
      }
      event "User defined": Value Change {
        n356 = event-data() -> ("NewVal"=w568:string)  [unwired: 6 out]
        n357 = local read "Recall Cluster"() -> (w569:T1)
        n358 = Bundle By Name(cluster=w569, "user defined"=w568) -> (w567:T1)
        n359 = local write "Recall Cluster"(w567) -> ()
      }
      event "Add2": Value Change {
        n360 = event-data() -> ()  [unwired: 7 out]
        n361 = case shown="True" "Add2" {
          frame False {
          }
          frame True {
            n362 = local read "Recall Cluster"() -> (w575:T1)
            n363 = Unbundle By Name(w575) -> ("Curve Names"=w576:string[])
            n364 = local read "Path Info"() -> (w571:u16)
            n365 = call "CRYAdd curve name.vi"("add/rename?"=TRUE, "Curve Names in"=w576) -> ("Curve Names out"=w572:string[])  [unwired: 9 in]
            n366 = case shown="1, Default" w571 {
              tunnel: w572 -> [w578 w579]
              frame 0 {
                n367 = local write "Specify Names"(w578) -> ()
              }
              frame 1, Default {
                n368 = local write "Auto Names"(w579) -> ()
              }
            }
            n369 = Build Array(w572) -> (w574:string[][])
            n370 = Transpose 2D Array(2D array=w574) -> (transposed array=w573:string[][])
            n371 = property on="Names Control" class="Tbl (strict)"("Val(Sgnl)"=w573) -> ()  [unwired: 2 in, 2 out]
          }
        }
      }
      event "Clear2": Value Change {
        n372 = event-data() -> ()  [unwired: 7 out]
        n373 = case shown="True" "Clear2" {
          frame False {
          }
          frame True {
            w584 = FALSE ("Sel_1")
            n374 = local read "Recall Cluster"() -> (w587:T1)
            n375 = Bundle By Name(cluster=w587, "Curves Selected?"=bool[] [], "Curve Names"=string[] []) -> (w582:T1)
            n376 = local write "Table change"(TRUE ("Table change")) -> ()
            n377 = local write "Recall Cluster"(w582) -> ()
            n378 = property on="Names Control" class="Tbl (strict)"("Value"=string[][] [] ("Table Control")) -> ()  [unwired: 2 in, 2 out]
            n379 = local write "Sel_1"(w584) -> ()
            n380 = local write "Sel_2"(w584) -> ()
            n381 = local write "Sel_3"(w584) -> ()
            n382 = local write "Sel_4"(w584) -> ()
            n383 = local write "Sel_5"(w584) -> ()
            n384 = local write "Sel_6"(w584) -> ()
          }
        }
      }
      event "Rename": Value Change {
        n385 = event-data() -> ()  [unwired: 7 out]
        n386 = case shown="True" "Rename" {
          frame False {
          }
          frame True {
            n387 = local read "Recall Cluster"() -> (w597:T1)
            n388 = local read "Current Row"() -> (w591:i32)
            n389 = Unbundle By Name(w597) -> ("Curve Names"=w598:string[])
            n390 = Greater Or Equal To 0?(x=w591) -> (x >= 0?=w592:bool)
            n391 = Select(t=w591, s=w592, f=0) -> (s? t:f=w589:i32)
            n392 = local read "Path Info"() -> (w593:u16)
            n393 = call "CRYAdd curve name.vi"("Curent Name"=w589, "add/rename?"=FALSE, "Curve Names in"=w598) -> ("Curve Names out"=w594:string[])  [unwired: 8 in]
            n394 = Build Array(w594) -> (w596:string[][])
            n395 = case shown="1, Default" w593 {
              tunnel: w594 -> [w600 w601]
              frame 0 {
                n396 = local write "Specify Names"(w600) -> ()
              }
              frame 1, Default {
                n397 = local write "Auto Names"(w601) -> ()
              }
            }
            n398 = Transpose 2D Array(2D array=w596) -> (transposed array=w595:string[][])
            n399 = property on="Names Control" class="Tbl (strict)"("Val(Sgnl)"=w595) -> ()  [unwired: 2 in, 2 out]
          }
        }
      }
      event "Format Value": Value Change {
        n400 = event-data() -> ()  [unwired: 7 out]
        n401 = case shown="True" "Format Value" {
          frame False {
          }
          frame True {
            n402 = flat-sequence {
              frame #0 {
                n403 = local read "Recall Cluster"() -> (w605:T1)
                n404 = Unbundle By Name(w605) -> ("format string.Lin Format String out"=w610:string)
                n405 = call "CRYRead format string.vi"("Format string"=w610) -> ("Notation"=w606:u16, "Digits"=w607:u16, "Precision"=w608:u16, "Hide Traling Zeros"=w609:bool)  [unwired: 7 in]
                n406 = call "CRYNumber Format.vi"("Notation"=w606, "Digits"=w607, "Precision"=w608, "Hide Trailing Zeros"=w609) -> ("Format string"=w604:string)  [unwired: 7 in]
                n407 = Bundle By Name(cluster=w605, "format string.Lin Format String out"=w604) -> (w603:T1)
                n408 = local write "Recall Cluster"(w603) -> ()
              }
              frame #1 {
                n409 = property on="Axis" class="Slide (strict)"() -> ("Value"=w611:u16)  [unwired: 2 in, 2 out]
                n410 = property on="Axis" class="Slide (strict)"("Val(Sgnl)"=w611) -> ()  [unwired: 2 in, 2 out]
              }
            }
          }
        }
      }
      event "Help": Value Change {
        n411 = event-data() -> ("NewVal"=w613:string)  [unwired: 6 out]
        n412 = local read "Recall Cluster"() -> (w614:T1)
        n413 = Bundle By Name(cluster=w614, "Help"=w613) -> (w612:T1)
        n414 = local write "Recall Cluster"(w612) -> ()
      }
      event "Main Tab": Value Change {
        n415 = event-data() -> ("NewVal"=w616:enum32{"Setting", "Help"})  [unwired: 6 out]
        n416 = local read "Recall Cluster"() -> (w617:T1)
        n417 = Bundle By Name(cluster=w617, "Tab Value"=w616) -> (w615:T1)
        n418 = local write "Recall Cluster"(w615) -> ()
      }
      event "Select All": Value Change {
        n419 = event-data() -> ("NewVal"=w625:bool)  [unwired: 6 out]
        n420 = local read "Recall Cluster"() -> (w622:T1)
        n421 = Unbundle By Name(w622) -> ("Curve Names"=w620:string[])
        n422 = Not(x=w625) -> (.not. x?=w624:bool)
        n423 = Array Size(array=w620) -> (size(s)=w623:i32)
        n424 = Initialize Array(w624, w623) -> (w621:bool[])
        n425 = local write "Table change"(TRUE ("Table change")) -> ()
        n426 = Bundle By Name(cluster=w622, "Curves Selected?"=w621) -> (w619:T1)
        n427 = local write "Recall Cluster"(w619) -> ()
      }
      event "Names Control": Value Change {
        n428 = event-data() -> ("NewVal"=w627:string[][])  [unwired: 6 out]
        n429 = local read "Recall Curve"() -> (w626:u16)
        n430 = case shown="0, Default" w626 {
          tunnel: w627 -> [w638 _]
          tunnel: w626 -> [_ _]
          frame 0, Default {
            # "Selection"
            n431 = local read "Recall Cluster"() -> (w636:T1)
            n432 = Index Array(array=w638, index (col)=0 ("disabled index (col)")) -> (element=w630:string[])  [unwired: 1 in]
            n433 = Array Size(array=w630) -> (size(s)=w633:i32)
            n434 = Unbundle By Name(w636) -> ("Curves Selected?"=w632:bool[])
            n435 = Array Size(array=w632) -> (size(s)=w634:i32)
            n436 = Greater?(x=w633, y=w634) -> (0:w635:bool)
            n437 = case shown="True" w635 {
              tunnel: w634 -> [_ w646]
              tunnel: w633 -> [_ w645]
              tunnel: w632 -> [w639 w643]
              tunnel: [w639 w641] -> w631
              frame False {
              }
              frame True {
                n438 = Subtract(x=w645, y=w646) -> (x-y=w644:i32)
                n439 = Initialize Array(TRUE ("element"), w644) -> (w642:bool[])
                n440 = Insert Into Array(array=w643, new element=w642) -> (w641:bool[])  [unwired: 1 in]
              }
            }
            n441 = local write "Table change"(TRUE ("Table change")) -> ()
            n442 = Bundle By Name(cluster=w636, "Curves Selected?"=w631, "Curve Names"=w630) -> (w629:T1)
            n443 = local write "Recall Cluster"(w629) -> ()
          }
          frame 1 {
            # "Last Only"
            n444 = local write "Table change"(FALSE ("Table change")) -> ()
          }
        }
      }
      event "Names Control": Mouse Down {
        n445 = event-data() -> ()  [unwired: 9 out]
        n446 = property on="Names Control" class="Tbl (strict)"() -> ("EditPos"=w648:T10)  [unwired: 2 in, 2 out]
        n447 = Unbundle By Name(w648) -> ("Row"=w649:i32)
        n448 = local write "Current Row"(w649) -> ()
      }
      event "Sel_1": Value Change {
        n449 = event-data() -> ("NewVal"=w655:bool)  [unwired: 6 out]
        n450 = local read "Recall Cluster"() -> (w654:T1)
        n451 = local read "Row"() -> (w652:u32)
        n452 = Unbundle By Name(w654) -> ("Curves Selected?"=w656:bool[])
        n453 = Replace Array Subset(array=w656, new element=w655, index=w652) -> (w653:bool[])
        n454 = Bundle By Name(cluster=w654, "Curves Selected?"=w653) -> (w651:T1)
        n455 = local write "Table change"(TRUE ("Table change")) -> ()
        n456 = local write "Recall Cluster"(w651) -> ()
      }
      event "Sel_2": Value Change {
        n457 = event-data() -> ("NewVal"=w665:bool)  [unwired: 6 out]
        n458 = local read "Recall Cluster"() -> (w667:T1)
        n459 = Unbundle By Name(w667) -> ("Curves Selected?"=w668:bool[], "Curve Names"=w658:string[])
        n460 = local read "Row"() -> (w662:u32)
        n461 = Array Size(array=w658) -> (size(s)=w660:i32)
        n462 = Greater Or Equal?(x=w660, y=2) -> (x >= y?=w657:bool)
        n463 = Add(x=w662, y=u32 1) -> (x+y=w664:u32)
        n464 = case shown="True" w657 {
          frame False {
          }
          frame True {
            n465 = local write "Table change"(TRUE ("Table change")) -> ()
          }
        }
        n466 = Replace Array Subset(array=w668, new element=w665, index=w664) -> (w666:bool[])
        n467 = Bundle By Name(cluster=w667, "Curves Selected?"=w666) -> (w661:T1)
        n468 = local write "Recall Cluster"(w661) -> ()
      }
      event "Sel_3": Value Change {
        n469 = event-data() -> ("NewVal"=w676:bool)  [unwired: 6 out]
        n470 = local read "Recall Cluster"() -> (w680:T1)
        n471 = Unbundle By Name(w680) -> ("Curves Selected?"=w681:bool[], "Curve Names"=w670:string[])
        n472 = local read "Row"() -> (w675:u32)
        n473 = Array Size(array=w670) -> (size(s)=w673:i32)
        n474 = Greater Or Equal?(x=w673, y=3) -> (x >= y?=w671:bool)
        n475 = Add(x=w675, y=u32 2) -> (x+y=w678:u32)
        n476 = case shown="True" w671 {
          frame False {
          }
          frame True {
            n477 = local write "Table change"(TRUE ("Table change")) -> ()
          }
        }
        n478 = Replace Array Subset(array=w681, new element=w676, index=w678) -> (w679:bool[])
        n479 = Bundle By Name(cluster=w680, "Curves Selected?"=w679) -> (w674:T1)
        n480 = local write "Recall Cluster"(w674) -> ()
      }
      event "Sel_4": Value Change {
        n481 = event-data() -> ("NewVal"=w690:bool)  [unwired: 6 out]
        n482 = local read "Recall Cluster"() -> (w693:T1)
        n483 = Unbundle By Name(w693) -> ("Curves Selected?"=w694:bool[], "Curve Names"=w683:string[])
        n484 = local read "Row"() -> (w688:u32)
        n485 = Array Size(array=w683) -> (size(s)=w686:i32)
        n486 = Greater Or Equal?(x=w686, y=4) -> (x >= y?=w684:bool)
        n487 = case shown="True" w684 {
          frame False {
          }
          frame True {
            n488 = local write "Table change"(TRUE ("Table change")) -> ()
          }
        }
        n489 = Add(x=w688, y=u32 3) -> (x+y=w691:u32)
        n490 = Replace Array Subset(array=w694, new element=w690, index=w691) -> (w692:bool[])
        n491 = Bundle By Name(cluster=w693, "Curves Selected?"=w692) -> (w687:T1)
        n492 = local write "Recall Cluster"(w687) -> ()
      }
      event "Sel_5": Value Change {
        n493 = event-data() -> ("NewVal"=w702:bool)  [unwired: 6 out]
        n494 = local read "Recall Cluster"() -> (w706:T1)
        n495 = Unbundle By Name(w706) -> ("Curves Selected?"=w707:bool[], "Curve Names"=w696:string[])
        n496 = Array Size(array=w696) -> (size(s)=w699:i32)
        n497 = local read "Row"() -> (w701:u32)
        n498 = Greater Or Equal?(x=w699, y=5) -> (x >= y?=w697:bool)
        n499 = case shown="True" w697 {
          frame False {
          }
          frame True {
            n500 = local write "Table change"(TRUE ("Table change")) -> ()
          }
        }
        n501 = Add(x=w701, y=u32 4) -> (x+y=w704:u32)
        n502 = Replace Array Subset(array=w707, new element=w702, index=w704) -> (w705:bool[])
        n503 = Bundle By Name(cluster=w706, "Curves Selected?"=w705) -> (w700:T1)
        n504 = local write "Recall Cluster"(w700) -> ()
      }
      event "Sel_6": Value Change {
        n505 = event-data() -> ("NewVal"=w715:bool)  [unwired: 6 out]
        n506 = local read "Recall Cluster"() -> (w719:T1)
        n507 = Unbundle By Name(w719) -> ("Curves Selected?"=w720:bool[], "Curve Names"=w709:string[])
        n508 = local read "Row"() -> (w714:u32)
        n509 = Array Size(array=w709) -> (size(s)=w712:i32)
        n510 = Greater Or Equal?(x=w712, y=6) -> (x >= y?=w710:bool)
        n511 = Add(x=w714, y=u32 5) -> (x+y=w717:u32)
        n512 = case shown="True" w710 {
          frame False {
          }
          frame True {
            n513 = local write "Table change"(TRUE ("Table change")) -> ()
          }
        }
        n514 = Replace Array Subset(array=w720, new element=w715, index=w717) -> (w718:bool[])
        n515 = Bundle By Name(cluster=w719, "Curves Selected?"=w718) -> (w713:T1)
        n516 = local write "Recall Cluster"(w713) -> ()
      }
    }
    n517 = property on="Names Control" class="Tbl (strict)"() -> ("Index Values"=w44:T5)  [unwired: 2 in, 2 out]
    n518 = local read "Row"() -> (w42:u32)
    n519 = Unbundle By Name(w44) -> ("Row"=w41:u32)
    n520 = global read "CRYMain Sub Window Global.vi" "gStop"() -> (w47:bool)
    n521 = Not Equal?(x=w41, y=w42) -> (x != y?=w43:bool)
    n522 = Or(x=w47, y="stop") -> (x .or. y?=w46:bool)
    n523 = Bundle("Apply"="Apply", "Load Test"="Load Test", w43, "Table change"="Table change", "Add Lib"="Add Lib", "OK"="OK", "Cancel"="Cancel") -> (w51:T11)  [unwired: 1 out]
    n524 = Cluster To Array(cluster=w51) -> (array=w50:bool[])
    n525 = Search 1D Array(1D array=w50, element=TRUE) -> (index of element=w48:i32)  [unwired: 1 out]
    n526 = case shown="4" w48 {
      tunnel: w41 -> [_ _ _ w138 _ _ _ _]
      tunnel: w37 -> [_ w54 _ _ _ _ _ _]
      frame Default {
      }
      frame 0 {
        n527 = global read "CRYMainGlobal.vi" "Access Level"() -> (w53:enum16{"Engineer", "Technician", "Operator"})
        n528 = case shown="\"Engineer\"" w53 {
          tunnel: w54 -> [w55 _]
          frame "Engineer" {
            n529 = flat-sequence {
              tunnel: [w58] -> w56
              tunnel: w55 -> [w57]
              tunnel: w56 -> [w64]
              frame #0 {
                n530 = local read "Recall Cluster"() -> (w58:T1)
                n531 = call "CRYFlatten Recall.vi"("Recall"=w58) -> ("Recall flattened"=w62:string)  [unwired: 10 in]
                n532 = call "CRYGet Current TS Steps.vi"() -> ("SelectStepNumber in Tree"=w59:i32, "Steps"=w60:T4[])  [unwired: 1 in, 9 out]
                n533 = Index Array(array=w60, index=w59) -> (element=w63:T4)
                n534 = Bundle By Name(cluster=w63, "Seq setup flattened"=w62) -> (w61:T4)
                n535 = call "CRYRecall.vi"("Setup in"=w61, "Step name"=w57) -> ()  [unwired: 9 in, 5 out]
              }
              frame #1 {
                n536 = local read "Path Info"() -> (w67:u16)
                n537 = Equal?(x=w67, y=u16 1) -> (x = y?=w65:bool)
                n538 = case shown="True" w65 {
                  tunnel: w67 -> [w71 _]
                  tunnel: [w70 w75] -> w68
                  frame False {
                    n539 = global read "CRYRecall Global.vi" "Recall Path"() -> (w72:path)
                    n540 = Path To String(path=w72) -> (string=w70:string)
                    n541 = local write "Base Path"(w72) -> ()
                    n542 = case shown="1, Default" w71 {
                      tunnel: w70 -> [w73 w74]
                      frame 0 {
                        n543 = local write "Specify Path"(w73) -> ()
                      }
                      frame 1, Default {
                        n544 = local write "Auto Path"(w74) -> ()
                      }
                    }
                  }
                  frame True {
                    n545 = local read "Base Path"() -> (w76:path)
                    n546 = Path To String(path=w76) -> (string=w75:string)
                  }
                }
                n547 = Bundle By Name(cluster=w64, "filepath"=w68) -> (w69:T1)
                n548 = local write "Recall Cluster"(w69) -> ()
              }
            }
          }
          frame "Operator", Default {
            n549 = call "CRYGet Error Message.vi"("Kind"="Step Setup") -> ("Window Title"=w78:string)  [unwired: 5 in, 5 out]
            n550 = call "CRYGet Access Level Message.vi"() -> ("Multibyte string"=w80:string)  [unwired: 11 in]
            n551 = call "CRYMessage Dialog.vi"("Window Title"=w78, "YesNoCancel"=T7."OK", "Message Content"=w80) -> ()  [unwired: 7 in, 2 out]
          }
        }
      }
      frame 1 {
        n552 = flat-sequence {
          frame #0 {
            n553 = local read "Recall Cluster"() -> (w98:T1)
            n554 = Unbundle By Name(w98) -> ("Name"=w112:string, "filepath"=w99:string, "all or last"=w94:i32, "File Path Mode"=w107:u16, "Curve Names"=w91:string[], "Template"=w106:u16[], "Axis"=w103:u16, "*.imp Path"=w102:path, "Filepath option"=w90:i16, "user defined"=w105:string, "Curves Selected?"=w95:bool[], "Help"=w101:string, "Tab Value"=w100:enum32{"Setting", "Help"}, "Selector"=w93:i32, "Use Default"=w92:bool, "Name"=w86:string, "Axis"=w85:u16)  [unwired: 2 out]
            n555 = property on="Value" class="Ring (strict)"() -> ("Strings []"=w113:string[])  [unwired: 2 in, 2 out]
            n556 = call "CRYGet Curve Library Data Name.vi"("sAction"="GetNameByType", "Type"=enum16{"Curves", "Values", "Results", "WFM"}."Values") -> ("sNames"=w87:string[])  [unwired: 6 in, 3 out]
            n557 = local write "User defined"(w105) -> ()
            n558 = Search 1D Array(1D array=w113, element=w112) -> (index of element=w108:i32)  [unwired: 1 in]
            n559 = local write "Axis"(w103) -> ()
            n560 = local write "Selector"(w93) -> ()
            n561 = local write "Use default"(w92) -> ()
            n562 = Search 1D Array(1D array=w87, element=w86) -> (index of element=w82:i32)  [unwired: 1 in]
            n563 = Equal?(x=w108, y=-1) -> (x = y?=w110:bool)
            n564 = local write ".imp Path"(w102) -> ()
            n565 = Less Than 0?(x=w82) -> (x < 0?=w84:bool)
            n566 = property on="File Path Mode" class="Slide (strict)"("Value"=w107) -> ()  [unwired: 2 in, 2 out]
            n567 = property on="Recall Curve" class="Slide (strict)"("Value"=w94) -> ()  [unwired: 2 in, 2 out]
            n568 = Select(t=0 ("y"), s=w110, f=w108) -> (s? t:f=w104:i32)
            n569 = property on="Temp" class="Arr (strict)"("Value"=w106) -> ()  [unwired: 2 in, 2 out]
            n570 = Select(t=0, s=w84, f=w82) -> (s? t:f=w83:i32)
            n571 = property on="Value" class="Ring (strict)"("Val(Sgnl)"=w104) -> ()  [unwired: 2 in, 2 out]
            n572 = flat-sequence {
              tunnel: w83 -> [w114]
              tunnel: w85 -> [w115]
              frame #0 {
                n573 = local write "Value"(w114) -> ()
              }
              frame #1 {
                n574 = property on="Axis" class="Slide (strict)"("Val(Sgnl)"=w115) -> ()  [unwired: 2 in, 2 out]
              }
            }
            n575 = Array Size(array=w91) -> (size(s)=w97:i32)
            n576 = property on="Help" class="Str"("Value"=w101) -> ()  [unwired: 2 in, 2 out]
            n577 = Equal To 0?(x=w97) -> (x = 0?=w96:bool)
            n578 = flat-sequence {
              tunnel: w99 -> [w120]
              tunnel: w96 -> [w119]
              tunnel: w95 -> [w118]
              tunnel: w91 -> [w117]
              tunnel: w90 -> [w116]
              tunnel: w90 -> [w129]
              frame #0 {
                n579 = case shown="True" w119 {
                  tunnel: w116 -> [w123 _]
                  tunnel: w120 -> [w121 _]
                  tunnel: w117 -> [w122 _]
                  tunnel: w118 -> [_ _]
                  frame False {
                    n580 = case shown="1, Default" w123 {
                      tunnel: w122 -> [w126 w128]
                      tunnel: w121 -> [w125 w127]
                      frame 0 {
                        n581 = local write "Specify Names"(w126) -> ()
                        n582 = local write "Specify Path"(w125) -> ()
                      }
                      frame 1, Default {
                        n583 = local write "Auto Names"(w128) -> ()
                        n584 = local write "Auto Path"(w127) -> ()
                      }
                    }
                    n585 = local write "Row"(u32 0 ("Row")) -> ()
                  }
                  frame True {
                  }
                }
              }
              frame #1 {
                n586 = property on="Path Info" class="Slide (strict)"("Val(Sgnl)"=w129) -> ()  [unwired: 2 in, 2 out]
              }
            }
            n587 = property on="Main Tab" class="TabCtl (strict)"("Value"=w100) -> ()  [unwired: 2 in, 2 out]
          }
          frame #1 {
            n588 = control-ref of="Board Tab"() -> (w131:refnum<vi>)
            n589 = control-ref of="This VI"() -> (w130:refnum<vi>)
            n590 = call "CRYAlign Steps VI Center.vi"("Tab2"=w131, "Input/Output"=TRUE ("Preview"), "VIRef"=w130) -> ()  [unwired: 1 in, 8 out]
          }
          frame #2 {
            n591 = local write "Load Test"(FALSE ("Load Test")) -> ()
            n592 = property on="Board Tab" class="TabCtl (strict)"("Visible"=TRUE) -> ()  [unwired: 2 in, 2 out]
          }
          frame #3 {
            n593 = local read "AddStep"() -> (w135:bool)
            n594 = local write "Add Lib"(w135) -> ()
          }
          frame #4 {
            n595 = local write "AddStep"(FALSE ("AddStep")) -> ()
          }
        }
      }
      frame 2 {
        n596 = flat-sequence {
          tunnel: w138 -> [w139]
          tunnel: [w139] -> w137
          tunnel: w137 -> [w150]
          frame #0 {
            n597 = local read "Recall Cluster"() -> (w141:T1)
            n598 = Unbundle By Name(w141) -> ("Curve Names"=w140:string[], "Curves Selected?"=w142:bool[])
            n599 = call "CRYRecall Curves Select.vi"("Curve Names"=w140, "Curves Selected?"=w142, "Row"=w139) -> ("Table Control"=w149:string[][], "Sel_1"=w148:bool, "Sel_2"=w147:bool, "Sel_3"=w146:bool, "Sel_4"=w145:bool, "Sel_6"=w143:bool, "Sel_5"=w144:bool)  [unwired: 6 in]
            n600 = local write "Names Control"(w149) -> ()
            n601 = local write "Sel_1"(w148) -> ()
            n602 = local write "Sel_2"(w147) -> ()
            n603 = local write "Sel_3"(w146) -> ()
            n604 = local write "Sel_4"(w145) -> ()
            n605 = local write "Sel_5"(w144) -> ()
            n606 = local write "Sel_6"(w143) -> ()
          }
          frame #1 {
            n607 = local write "Row"(w150) -> ()
          }
        }
      }
      frame 3 {
        n608 = local read "Recall Cluster"() -> (w153:T1)
        n609 = Unbundle By Name(w153) -> ("Curve Names"=w152:string[], "Curves Selected?"=w154:bool[])
        n610 = local read "Row"() -> (w162:u32)
        n611 = local write "Table change"(FALSE ("Table change")) -> ()
        n612 = call "CRYRecall Curves Select.vi"("Curve Names"=w152, "Curves Selected?"=w154, "Row"=w162) -> ("Table Control"=w161:string[][], "Sel_1"=w160:bool, "Sel_2"=w159:bool, "Sel_3"=w158:bool, "Sel_4"=w157:bool, "Sel_6"=w155:bool, "Sel_5"=w156:bool)  [unwired: 6 in]
        n613 = local write "Names Control"(w161) -> ()
        n614 = local write "Sel_1"(w160) -> ()
        n615 = local write "Sel_2"(w159) -> ()
        n616 = local write "Sel_3"(w158) -> ()
        n617 = local write "Sel_4"(w157) -> ()
        n618 = local write "Sel_5"(w156) -> ()
        n619 = local write "Sel_6"(w155) -> ()
      }
      frame 4 {
        n620 = flat-sequence {
          frame #0 {
            n621 = local read "Recall Cluster"() -> (w169:T1)
            n622 = call "CRYGet Current TS Steps.vi"() -> ("SelectStepNumber in Tree"=w165:i32, "Steps"=w164:T4[])  [unwired: 7 in, 3 out]
            n623 = local read "Data type"() -> (w170:string)
            n624 = call "CRYFlatten Recall.vi"("Recall"=w169) -> ("Recall flattened"=w167:string)  [unwired: 10 in]
            n625 = Index Array(array=w164, index=w165) -> (element=w168:T4)
            n626 = call "CRYRecall Curve Name Replace.vi"("Data type"=w170, "Setup in"=w168, "Step setup In"=w167, "sOption1"="AddStep") -> ()  [unwired: 8 in]
          }
          frame #1 {
            n627 = global read "CRYStepSetup Global.vi" "Load from AddStep"() -> (w172:bool)
            n628 = local read "Proper VI No"() -> (w171:i32)
            n629 = local write "Add Lib"(FALSE ("Add Lib")) -> ()
            n630 = case shown="True" w172 {
              tunnel: w171 -> [_ w175]
              frame False {
              }
              frame True {
                n631 = global write "CRYStepSetup Global.vi" "Load from AddStep"(FALSE ("Load from AddStep")) -> ()
                n632 = call "CRYStepData Manipulate.vi"("sAction"="Backup", "StepNo."=w175) -> ()  [unwired: 10 in]
              }
            }
          }
        }
        n633 = local write "Table change"(TRUE ("Table change")) -> ()
      }
      frame 5 {
        n634 = flat-sequence {
          frame #0 {
            n635 = global read "CRYMainGlobal.vi" "Access Level"() -> (w178:enum16{"Engineer", "Technician", "Operator"})
            n636 = case shown="\"Technician\", Default" w178 {
              frame "Engineer" {
                n637 = flat-sequence {
                  tunnel: [w181] -> w179
                  tunnel: w179 -> [w187]
                  frame #0 {
                    n638 = local read "Recall Cluster"() -> (w186:T1)
                    n639 = local read "Proper VI No"() -> (w182:i32)
                    n640 = call "CRYFlatten Recall.vi"("Recall"=w186) -> ("Recall flattened"=w181:string)  [unwired: 10 in]
                    n641 = local write "Table change"(TRUE ("Table change")) -> ()
                    n642 = call "CRYPreUpdate Sequence.vi"("EventName"="SequenceUpdate", "Proper VI No"=w182, "Project View Step Name Identifier Arg1"="", "Step flattened Arg2"=w181, "AllChangeFlg"=TRUE ("Name/Identifier")) -> ()  [unwired: 11 in]
                  }
                  frame #1 {
                    n643 = call "CRYGet Current TS Steps.vi"() -> ("SelectStepNumber in Tree"=w189:i32, "Steps"=w188:T4[])  [unwired: 7 in, 3 out]
                    n644 = local read "Data type"() -> (w192:string)
                    n645 = Index Array(array=w188, index=w189) -> (element=w191:T4)
                    n646 = call "CRYRecall Curve Name Replace.vi"("Data type"=w192, "Setup in"=w191, "Step setup In"=w187, "sOption1"="StepOK") -> ()  [unwired: 8 in]
                  }
                }
              }
              frame "Technician", Default {
                n647 = call "CRYGet Error Message.vi"("Kind"="Step Setup") -> ("Window Title"=w195:string)  [unwired: 5 in, 5 out]
                n648 = call "CRYGet Access Level Message.vi"("sAction"="OK") -> ("Multibyte string"=w197:string)  [unwired: 10 in]
                n649 = call "CRYMessage Dialog.vi"("Window Title"=w195, "YesNoCancel"=T7."OK", "Message Content"=w197) -> ()  [unwired: 7 in, 2 out]
              }
            }
          }
          frame #1 {
            n650 = local write "OK"(FALSE ("OK")) -> ()
          }
        }
        n651 = local write "stop"(TRUE ("stop")) -> ()
      }
      frame 6 {
        n652 = flat-sequence {
          frame #0 {
            n653 = local read "Proper VI No"() -> (w200:i32)
            n654 = call "CRYStepData Manipulate.vi"("sAction"="Restore", "StepNo."=w200) -> ()  [unwired: 10 in]
          }
          frame #1 {
            n655 = local write "Cancel"(FALSE ("Cancel")) -> ()
          }
        }
        n656 = local write "stop"(TRUE ("stop")) -> ()
      }
    }
  }
  n657 = flat-sequence {
    tunnel: w3 -> [_]
    frame #0 {
      n658 = control-ref of="This VI"() -> (w722:refnum<vi>)
      n659 = call "CRYWork Before Step Close.vi"("StepVI Ref"=w722) -> ()  [unwired: 11 in]
    }
    frame #1 {
      n660 = local write "EndFlag"(TRUE ("EndFlag")) -> ()
    }
  }
